vi "Configure Results Names.vi"(8 "error in":errorcluster, 11 "DAC Traverse in":refnum<class "DAC Traverse.lvclass">) -> (0 "error out":errorcluster, 3 "DAC Traverse out":refnum<class "DAC Traverse.lvclass">)   [LabVIEW 2019, in "DAC.lvlib" / "DAC Traverse.lvclass"]
uses:
  DAC Traverse.lvclass
  DAC Traverse.lvclass/DAC Traverse.ctl
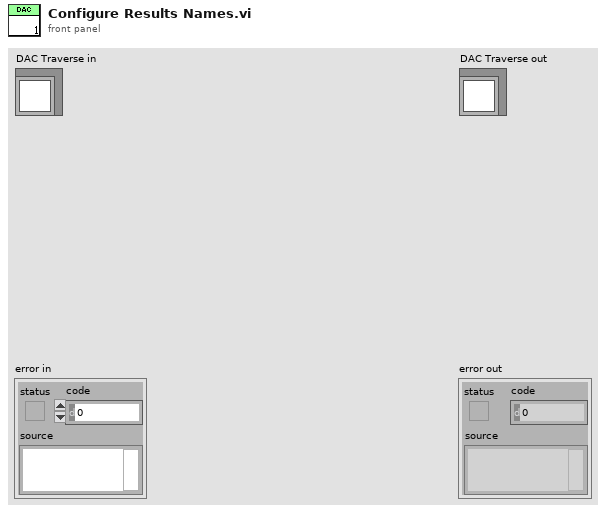
[diagram p1: front panel]
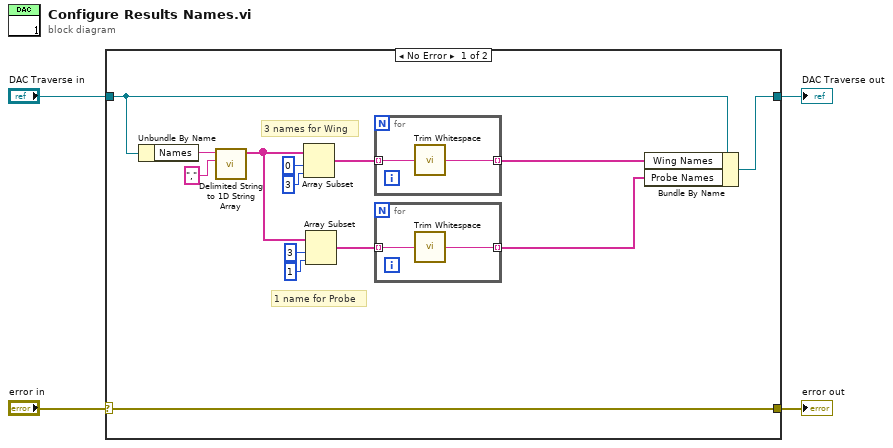
[diagram p0: block diagram]
diagram:
  n1 = case shown="No Error" "error in" {
    selector: "error in" -> [w18 w24]
    tunnel: [w18 w24] -> w3
    tunnel: [w17 w23] -> w1
    tunnel: "DAC Traverse in" -> [w16 w23]
    frame No Error {
      # "1 name for Probe"
      # "3 names for Wing"
      n2 = Unbundle By Name(w16) -> ("Names"=w9:string)
      n3 = call <vilib>:"Delimited String to 1D String Array.vi"("delimiter"=",", "delimited string"=w9) -> ("string array"=w10:string[])  [unwired: 9 in]
      n4 = Array Subset(array=w10, index=0, length=3) -> (w8:string[])
      n5 = Array Subset(array=w10, index=3, length=1) -> (w6:string[])
      n6 = for {
        tunnel: w8 -> [w22] mode=indexing
        tunnel: [w21] -> w7 mode=indexing
        n7 = call <vilib>:"Trim Whitespace.vi"("string"=w22) -> ("trimmed string"=w21:string)  [unwired: 1 in]
      }
      n8 = for {
        tunnel: w6 -> [w20] mode=indexing
        tunnel: [w19] -> w5 mode=indexing
        n9 = call <vilib>:"Trim Whitespace.vi"("string"=w20) -> ("trimmed string"=w19:string)  [unwired: 1 in]
      }
      n10 = Bundle By Name(cluster=w16, "Wing Names"=w7, "Probe Names"=w5) -> (w17:refnum<class "DAC Traverse.lvclass">)
    }
    frame Error {
    }
  }
  "error out" <- w3
  "DAC Traverse out" <- w1
